vi "xcorr_packet.bkp.vi"(0 "x":u32, 1 "y":u32, 2 "width":u16) -> (8 "out":u64, 9 "valid":bool)   [LabVIEW 2017]
uses:
  <vilib>/rvi/FXPMathLib/basic elements/FxpDiscreteDelay/XNode/nifxpmath_DiscreteDelay.xnode
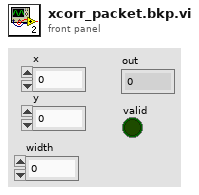
[diagram p1: front panel]
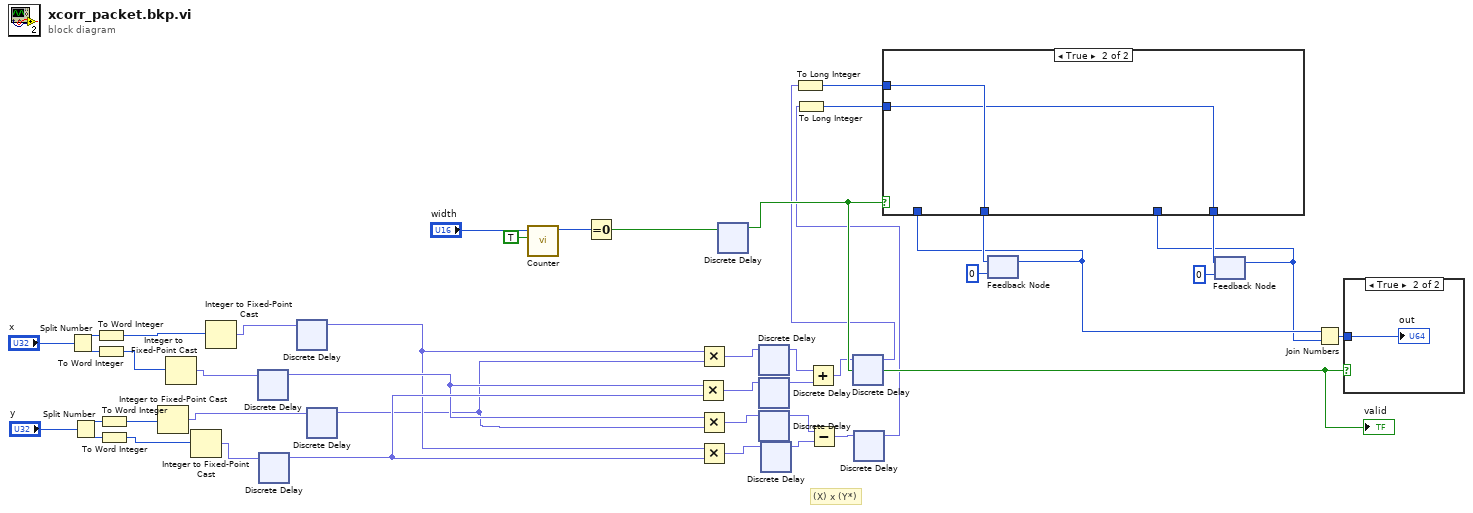
[diagram p0: block diagram]
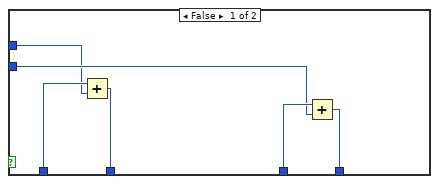
[diagram p3: hidden frame]
diagram:
  # "(X) x (Y*)"
  n1 = Split Number(x="x") -> (hi(x)=w30:u16, lo(x)=w31:u16)
  n2 = Split Number(x="y") -> (hi(x)=w32:u16, lo(x)=w33:u16)
  n3 = To Word Integer(number=w30) -> (16bit integer=w12:i16)
  n4 = To Word Integer(number=w31) -> (16bit integer=w13:i16)
  n5 = To Word Integer(number=w32) -> (16bit integer=w11:i16)
  n6 = To Word Integer(number=w33) -> (16bit integer=w27:i16)
  n7 = Integer to Fixed-Point Cast(integer=w11) -> (fixed-point=w8:fxp<+/-,16,16>)  [unwired: 1 in]
  n8 = Integer to Fixed-Point Cast(integer=w13) -> (fixed-point=w7:fxp<+/-,16,16>)  [unwired: 1 in]
  n9 = Integer to Fixed-Point Cast(integer=w27) -> (fixed-point=w10:fxp<+/-,16,16>)  [unwired: 1 in]
  n10 = Integer to Fixed-Point Cast(integer=w12) -> (fixed-point=w5:fxp<+/-,16,16>)  [unwired: 1 in]
  n11 = xnode "Discrete Delay"("D"=w7) -> ("Q"=w6:fxp<+/-,16,16>)
  n12 = xnode "Discrete Delay"("D"=w10) -> ("Q"=w9:fxp<+/-,16,16>)
  n13 = xnode "Discrete Delay"("D"=w5) -> ("Q"=w3:fxp<+/-,16,16>)
  n14 = xnode "Discrete Delay"("D"=w8) -> ("Q"=w2:fxp<+/-,16,16>)
  n15 = call "Counter.vi"("enable"=TRUE, "limit"="width") -> ("count"=w44:u16)  [unwired: 9 in]
  n16 = Equal To 0?(x=w44) -> (x = 0?=w26:bool)
  n17 = Multiply(x=w6, y=w9) -> (x*y=w19:fxp<+/-,32,32>)
  n18 = Multiply(x=w3, y=w2) -> (x*y=w18:fxp<+/-,32,32>)
  n19 = Multiply(x=w6, y=w2) -> (x*y=w20:fxp<+/-,32,32>)
  n20 = Multiply(x=w3, y=w9) -> (x*y=w21:fxp<+/-,32,32>)
  n21 = xnode "Discrete Delay"("D"=w26) -> ("Q"=w25:bool)
  "valid" <- w25
  n22 = xnode "Discrete Delay"("D"=w18) -> ("Q"=w14:fxp<+/-,32,32>)
  n23 = xnode "Discrete Delay"("D"=w19) -> ("Q"=w15:fxp<+/-,32,32>)
  n24 = xnode "Discrete Delay"("D"=w20) -> ("Q"=w16:fxp<+/-,32,32>)
  n25 = xnode "Discrete Delay"("D"=w21) -> ("Q"=w17:fxp<+/-,32,32>)
  n26 = Add(x=w14, y=w15) -> (x+y=w24:fxp<+/-,33,33>)
  n27 = Subtract(x=w16, y=w17) -> (x-y=w23:fxp<+/-,32,32>)
  n28 = xnode "Discrete Delay"("D"=w24) -> ("Q"=w4:fxp<+/-,33,33>)
  n29 = To Long Integer(number=w4) -> (32bit integer=w28:i32)
  n30 = xnode "Discrete Delay"("D"=w23) -> ("Q"=w22:fxp<+/-,32,32>)
  n31 = To Long Integer(number=w22) -> (32bit integer=w29:i32)
  n32 = feedback #1(0) -> (w38:i32)
  n33 = feedback #2(0) -> (w34:i32)
  n34 = case shown="True" w25 {
    tunnel: [w50 w52] -> w42
    tunnel: w38 -> [w49 _]
    tunnel: [w48 w51] -> w35
    tunnel: w34 -> [w47 _]
    tunnel: w29 -> [w46 w51]
    tunnel: w28 -> [w45 w52]
    frame False {
      n35 = Add(x=w49, y=w45) -> (x+y=w50:i32)
      n36 = Add(x=w47, y=w46) -> (x+y=w48:i32)
    }
    frame True {
    }
  }
  n37 = feedback-in #1(w42) -> ()
  n38 = feedback-in #2(w35) -> ()
  n39 = Join Numbers(hi=w38, lo=w34) -> ((hi.lo)=w37:u64)
  n40 = case shown="True" w25 {
    tunnel: w37 -> [_ w53]
    frame False {
    }
    frame True {
      "out" <- w53
    }
  }
